vi "Constrained Nonlinear Curve Fit.vi"   [LabVIEW 2017, in "NI_Gmath.lvlib"]
doc: "Uses either the Levenberg-Marquardt algorithm or the trust-region dogleg algorithm to determine the set of parameters that best fit the set of input data points (<B>X</B>, <B>Y</B>) as expressed by a nonlinear function y = <B>f(x,a)</B>, where a is the set of parameters. You must manually select the polymorphic instance to use."
uses:
  <vilib>/gmath/NI_Gmath.lvlib
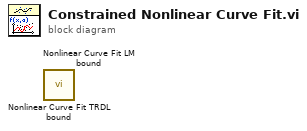
[diagram p0: block diagram]
diagram:
  n1 = call <vilib>:"Nonlinear Curve Fit TRDL bound.vi"() -> ()  [unwired: 10 in, 6 out]
  n2 = call <vilib>:"Nonlinear Curve Fit LM bound.vi"() -> ()  [unwired: 10 in, 6 out]
